vi "picoquant_split_channels.vi"(7 "acq_mode":T1=2 items=["T2"=2, "T3"=3], 8 "error in (no error)":errorcluster, 9 "sync":u64[](array[numeric]), 10 "channels":u8[](array[numeric]), 11 "times":u64[](array[numeric])) -> (0 "error out":errorcluster, 2 "ch2_array":u64[](array[numeric]), 3 "ch1_array":u64[](array[numeric]), 4 "ch2_tally":u64, 6 "ch1_tally":u64)   [LabVIEW 2015]
uses:
  picoquant_Tmodes.ctl
  lvoop_cfuncs/Debug/lvoop_cfuncs.dll
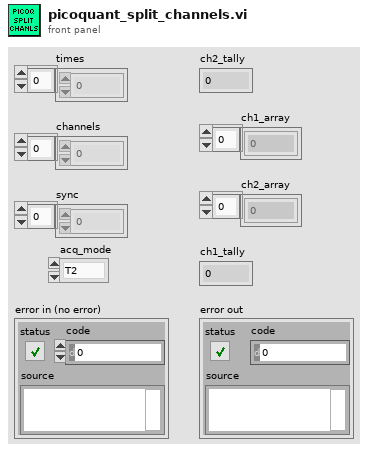
[diagram p1: front panel]
types:
  T1 = typedef "picoquant_Tmodes.ctl" = u16
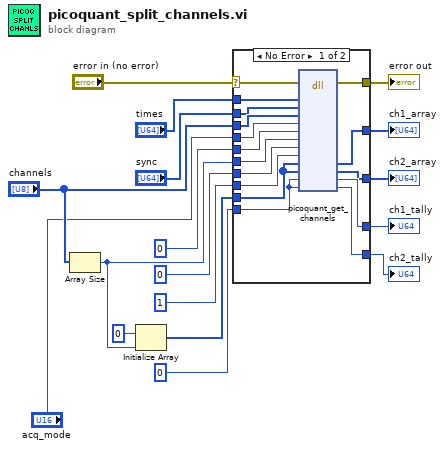
[diagram p0: block diagram]
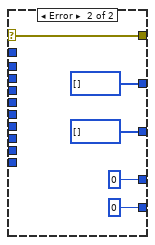
[diagram p2: hidden frame]
diagram:
  n1 = Array Size(array="channels") -> (size(s)=w10:i32)
  n2 = Initialize Array(u64 0, w10) -> (w12:u64[])
  n3 = case shown="No Error" "error in (no error)" {
    selector: "error in (no error)" -> [w19 w38]
    tunnel: [w33 u64 0 ("ch2_tally")] -> w17
    tunnel: [w32 u64 0 ("ch1_tally")] -> w16
    tunnel: [w31 u64[] [] ("ch2_array")] -> w15
    tunnel: [w30 u64[] [] ("ch1_array")] -> w14
    tunnel: u64 0 ("ch1_tally") -> [w29 _]
    tunnel: w12 -> [w28 _]
    tunnel: w10 -> [w27 _]
    tunnel: u8 1 ("ch2") -> [w26 _]
    tunnel: u8 0 ("ch1") -> [w25 _]
    tunnel: "channels" -> [w24 _]
    tunnel: u64 0 ("sync_period") -> [w23 _]
    tunnel: "acq_mode" -> [w22 _]
    tunnel: "sync" -> [w21 _]
    tunnel: "times" -> [w20 _]
    tunnel: [w18 w38] -> w2
    frame No Error {
      n4 = dll-call lib="C:/Users/MX-Microscope/Documents/LabVIEW Data/pcfs_lvoop_2017-master_170904/lvoop_dll-master/lvoop_cfuncs/Debug/lvoop_cfuncs.dll" fn="picoquant_get_channels"(error in=w19, "photon_times"=w20, "sync"=w21, "channels"=w24, "tmode"=w22, "sync_period"=w23, "num_records"=w27, "ch1"=w25, "ch2"=w26, "ch1_array"=w28, "ch2_array"=w28, "ch1_tally"=w29, "ch2_tally"=w29) -> (error out=w18:errorcluster, "ch1_array"=w30:u64[], "ch2_array"=w31:u64[], "ch1_tally"=w32:u64, "ch2_tally"=w33:u64)  [unwired: 11 in, 1 out]
    }
    frame Error {
    }
  }
  "error out" <- w2
  "ch2_tally" <- w17
  "ch1_tally" <- w16
  "ch2_array" <- w15
  "ch1_array" <- w14
